vi "ni579x EEPROM Byte Program.vi"(0 "Register Bus":T1, 1 "scope":string(combo)="characterization data eeprom", 5 "address":u32 format="%x", 7 "byte":u8 format="%x", 11 "Error In":errorcluster) -> (4 "Register Bus (out)":T1, 15 "Error Out":errorcluster)   [LabVIEW 2015, in "ni579x Config v2 Host.lvlib"]
uses:
  <instrlib>/ni579x/Config/v2/Host/ni579x Config v2 Host.lvlib
  <instrlib>/_niInstr/Register Bus/v0/Host/Public/Register Bus Session.ctl
  <instrlib>/_niInstr/Register Bus/v0/Host/Private/Session Data.ctl
  <instrlib>/ni579x/Config/v2/Shared/Types/ni579x FAM Register Offset.ctl
  <instrlib>/ni579x/Config/v2/Shared/Types/ni579x FAM Register Operation.ctl
  <instrlib>/ni579x/Config/v2/Shared/ni579x Config v2 Shared.lvlib
  <instrlib>/_niInstr/Register Bus/v0/Host/niInstr Register Bus v0 Host.lvlib
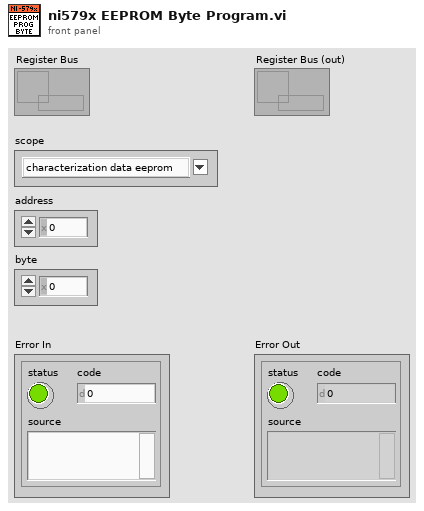
[diagram p1: front panel]
types:
  T1 = typedef "niInstr Register Bus v0 Host.lvlib/Register Bus Session.ctl" = refnum<queue>
  T2 = typedef "ni579x Config v2 Shared.lvlib/ni579x FAM Register Operation.ctl" = cluster{"FAM Register Offset":T3, "Address":u32, "Write (T)/Read (F)":bool, "Write Data":u32}
  T3 = typedef "ni579x Config v2 Shared.lvlib/ni579x FAM Register Offset.ctl" = u8
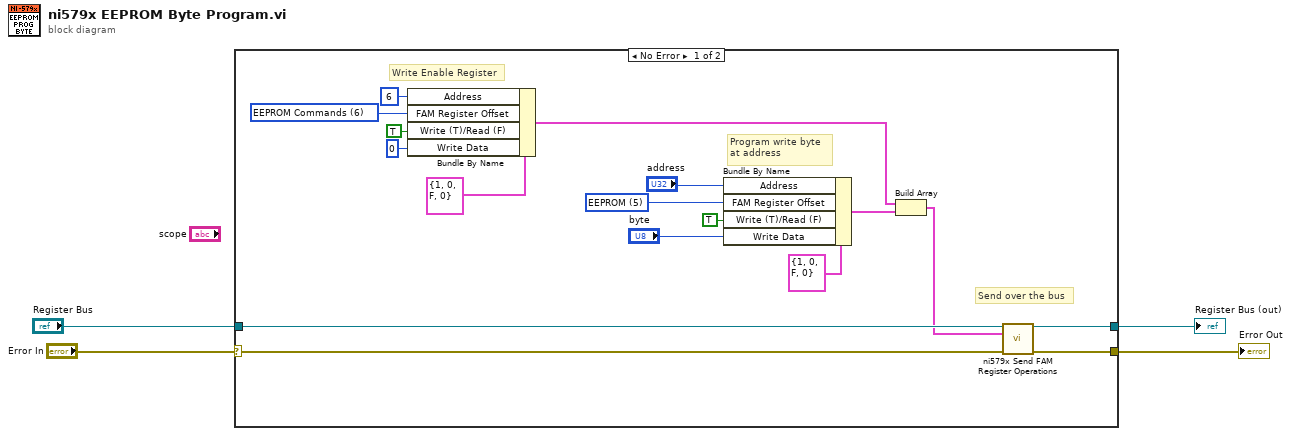
[diagram p0: block diagram]
diagram:
  n1 = case shown="No Error" "Error In" {
    selector: "Error In" -> [w18 w23]
    tunnel: [w20 w23] -> w3
    tunnel: "Register Bus" -> [w19 w22]
    tunnel: [w21 w22] -> w1
    frame No Error {
      w6 = T3 5 items=["ADC"=1, "DAC"=2, "Clock Distribution Chip"=3, "Frequency/Phase Adjust DAC"=4, "EEPROM"=5, "EEPROM Commands"=6, "LO1"=7, "Rx Atten Pre-LNA"=9, "Rx Atten Post-LNA"=10, "Tx Atten"=11] ("FAM Register Offset")
      w7 = T3 6 items=["ADC"=1, "DAC"=2, "Clock Distribution Chip"=3, "Frequency/Phase Adjust DAC"=4, "EEPROM"=5, "EEPROM Commands"=6, "LO1"=7, "Rx Atten Pre-LNA"=9, "Rx Atten Post-LNA"=10, "Tx Atten"=11] ("FAM Register Offset")
      # "Program write byte\nat address"
      # "Write Enable Register"
      # "Send over the bus"
      n2 = Bundle By Name(cluster=T2 {"FAM Register Offset"=1, "Address"=0, "Write (T)/Read (F)"=FALSE, "Write Data"=0} ("FAM Register Operation"), "Address"=u32 6, "FAM Register Offset"=w7, "Write (T)/Read (F)"=TRUE, "Write Data"=u32 0) -> (w13:T2)
      n3 = Bundle By Name(cluster=T2 {"FAM Register Offset"=1, "Address"=0, "Write (T)/Read (F)"=FALSE, "Write Data"=0} ("FAM Register Operation"), "Address"="address", "FAM Register Offset"=w6, "Write (T)/Read (F)"=TRUE, "Write Data"="byte") -> (w12:T2)
      n4 = Build Array(w13, w12) -> (w11:T2[])
      n5 = call <instrlib>:"ni579x Send FAM Register Operations.vi"("Register Bus"=w19, "FAM Register Operations"=w11, "Error In"=w18) -> ("Register Bus (out)"=w21:T1, "Error Out"=w20:errorcluster)  [unwired: 10 in, 1 out]
    }
    frame Error {
    }
  }
  "Register Bus (out)" <- w1
  "Error Out" <- w3
